vi "Halvorsen_Euler_Fast.vi"(0 "tolerance":dbl=1e-13, 1 "Error Analysis":u16(ring)=4 items=["Max", "Max_Norm", "Norm", "Last Value", "Last Constant"], 3 "Шаг h, с":dbl=0.01, 4 "k":i32=8, 5 "Время, с":dbl=30.0, 7 "Hmax":dbl=1.0, 8 "Parameters":dbl[](array[numeric])=[1.4, 1.4, 1.4], 10 "last_point_Thomas":dbl[](array[numeric])=[2.3727475682665875, 0.23609824454436878, 0.4447912442126299], 13 "Hmin":dbl=0.001, 15 "Points count":i32=2, 18 "n":i32[](array[numeric])=[1, 2, 3, 4, 5, 6, 7, 8, 18, 20, 22], 19 "Ext.Type":u16(ring) items=["FNode", "MathScript", "ECD8 Arrays", "ECD8 Fnode", "ECD8 FnodeDiv", "FNode Exp"]) -> (6 "Elapsed Time":dbl=0.8335924918947057, 12 "Number of steps":i32=29504, 14 "Error Estimation":dbl=9.972073185504694, 17 "Rejected steps":i32=56)   [LabVIEW 2016]
uses:
  <vilib>/Analysis/_algsub.llb/Real Vector Norm.vi
  <vilib>/Analysis/5stat.llb/RMS (DBL).vi
  <vilib>/Analysis/NI_AALBase.lvlib
  <vilib>/Analysis/NI_AALPro.lvlib
panel:
  in  "Initial Conditions":dbl[](array[numeric])=[1.0, 0.0, 1.0]
  out "Last Value Reference":dbl[](array[numeric])=[-8.132376937433255, -1.7681295405184005, -0.1250130264252919] format="%#_15f"
  out "Rejected Steps":i32[](graph)
  out "Last Value":dbl[](array[numeric])=[-7.1287069315310125, 0.8112482175083243, -2.527381111815407] format="%#_16f"
  out "Step time variation":dbl[](graph)=[0.8416094721687841, 0.8255755116206274]
  out "Real Error":dbl[][](graph)
  out "Step Variation":dbl[](graph)
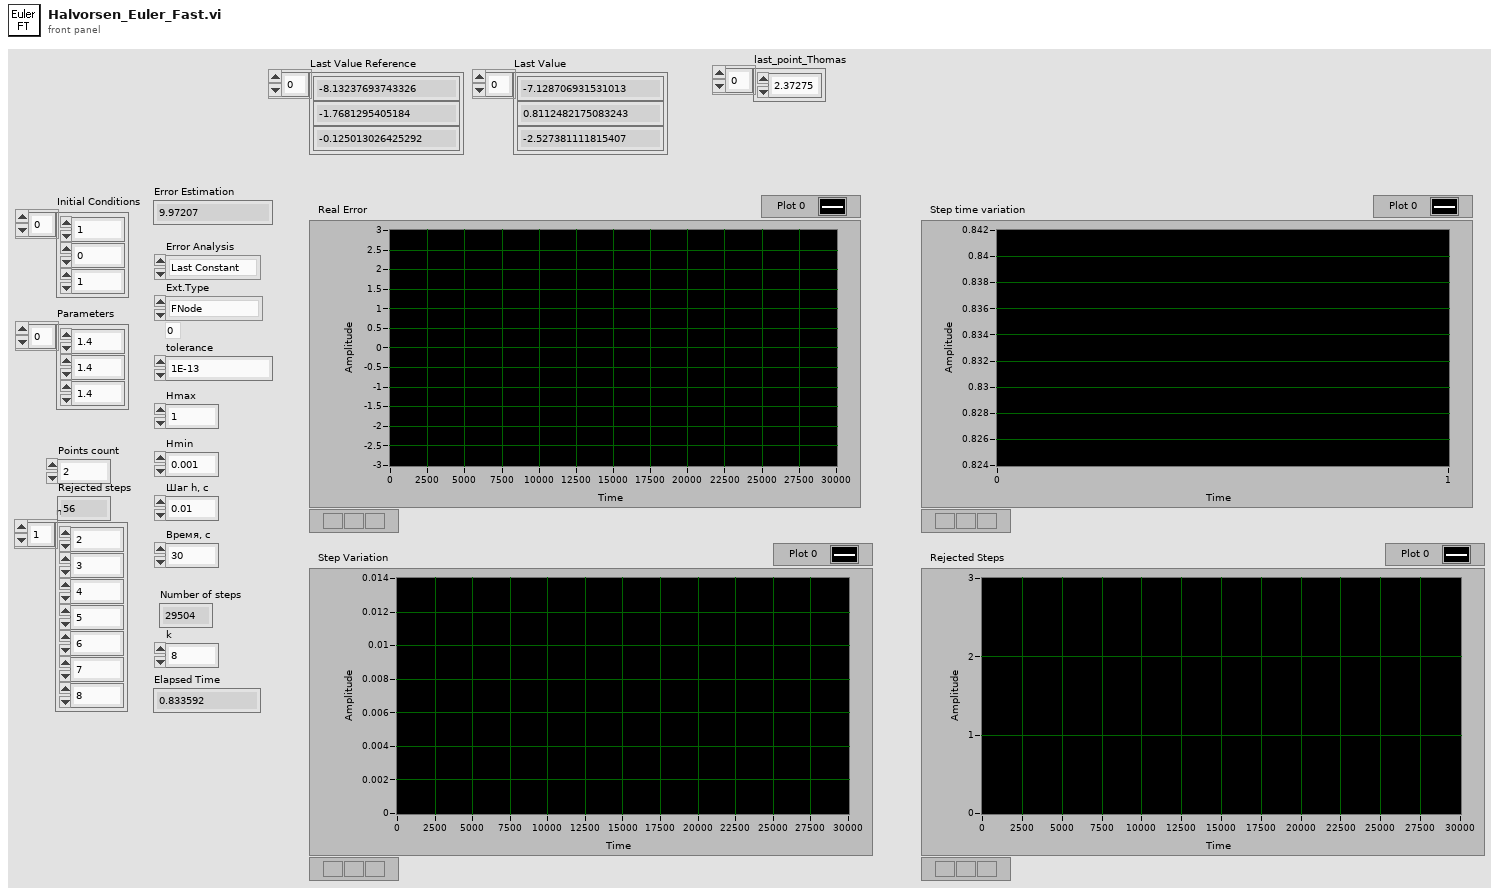
[diagram p1: front panel]
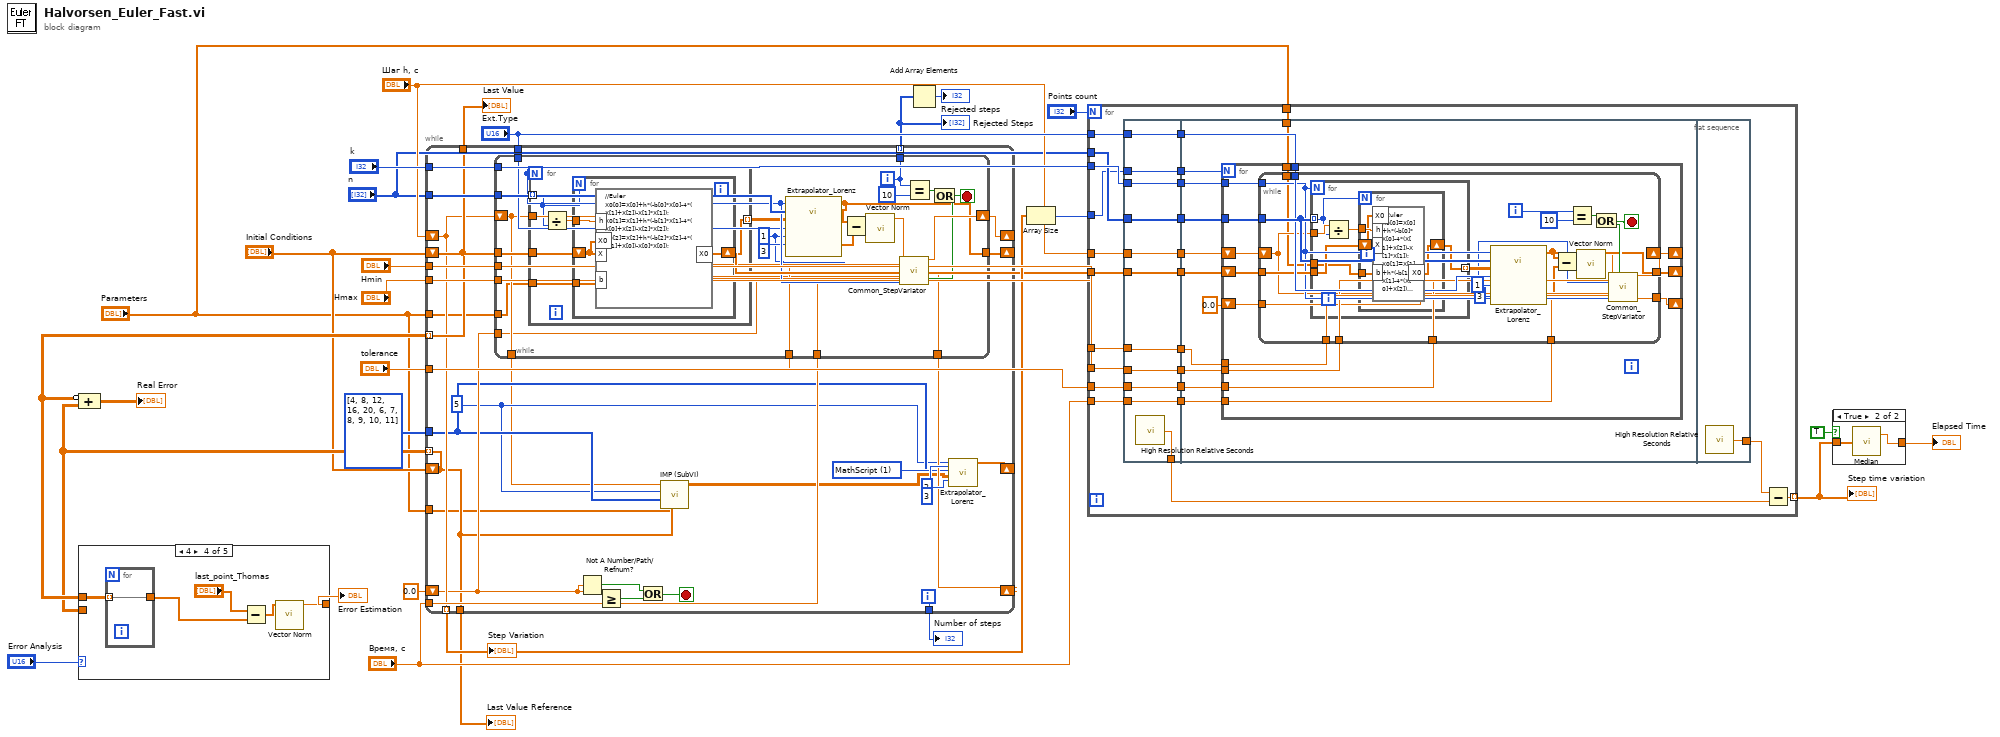
[diagram p0: block diagram]
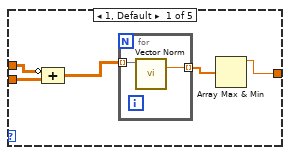
[diagram p2: hidden frame]
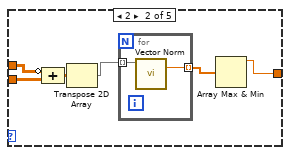
[diagram p3: hidden frame]
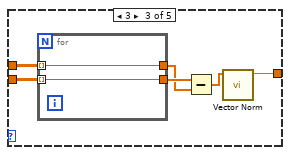
[diagram p4: hidden frame]
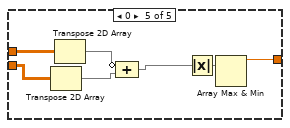
[diagram p5: hidden frame]
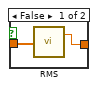
[diagram p6: hidden frame]
diagram:
  n1 = while {
    shift-right: [w50] -> _
    shift-left: "Initial Conditions" -> [w43]
    tunnel: "n" -> [w57]
    tunnel: "k" -> [w55]
    tunnel: "Ext.Type" -> [w46]
    shift-right: [w54] -> _
    shift-left: "Шаг h, с" -> [w37]
    shift-right: [w45] -> _
    shift-left: 0.0 -> [w36]
    tunnel: [w37] -> w13 mode=indexing
    tunnel: "Время, с" -> [w44]
    tunnel: [w56] -> w23
    tunnel: "tolerance" -> [w51]
    tunnel: "Hmin" -> [w53]
    tunnel: "Hmax" -> [w52]
    tunnel: [w43] -> w6 mode=indexing
    shift-right: [w49] -> _
    shift-left: "Initial Conditions" -> [w31]
    tunnel: i32[] [4, 8, 12, 16, 20, 6, 7, 8, 9, 10, 11] ("n 2") -> [w34]
    tunnel: [w31] -> w5 mode=indexing
    tunnel: [w43] -> w11
    tunnel: [w42] -> w10 mode=indexing
    tunnel: [w31] -> w4
    tunnel: "Parameters" -> [w35]
    tunnel: "Parameters" -> [w30]
    i -> [w56]
    stop <- w40 stop-if-true
    w41 = u16 1 items=["FNode", "MathScript", "ECD8 Arrays", "ECD8 Fnode", "ECD8 FnodeDiv"] ("Ext.Type")
    w33 = 5
    n2 = while {
      tunnel: w57 -> [w82]
      tunnel: w55 -> [w81]
      tunnel: w53 -> [w79]
      tunnel: w52 -> [w78]
      tunnel: w51 -> [w77]
      tunnel: [w60] -> w50
      tunnel: w46 -> [w74]
      tunnel: [w65] -> w45
      tunnel: w44 -> [w73]
      tunnel: w43 -> [w72]
      shift-right: [w80] -> w54
      shift-left: w37 -> [w67]
      tunnel: [w67] -> w32
      tunnel: [w66] -> w42
      tunnel: w36 -> [w64]
      tunnel: w35 -> [w62]
      i -> [w66]
      stop <- w69 stop-if-true
      w63 = 1 ("input variable")
      n3 = for {
        N: w81 -> [_]
        tunnel: w82 -> [w85] mode=indexing
        tunnel: w67 -> [w86]
        tunnel: w72 -> [w88]
        tunnel: [w87] -> w75 mode=indexing
        tunnel: w62 -> [w83]
        n4 = Divide(x=w86, y=w85) -> (x/y=w84:dbl)
        n5 = for {
          N: w85 -> [_]
          shift-right: [w92] -> w87
          shift-left: w88 -> [w90]
          tunnel: w84 -> [w91]
          tunnel: w83 -> [w89]
          n6 = formula code="//Euler\nX0[0]=X[0]+h*(-b[0]*X[0]-4*(X[1]+X[2])-X[1]*X[1]);\nX0[1]=X[1]+h*(-b[1]*X[1]-4*(X[0]+X[2])-X[2]*X[2]);\nX0[2]=X[2]+h*(-b[2]*X[2]-4*(X[1]+X[0])-X[0]*X[0]);"("X"=w90, "h"=w91, "X0"=w90, "b"=w89) -> ("X0"=w92:dbl[])
        }
      }
      n7 = call "Extrapolator_Lorenz.vi"("Порядок экстраполятора"=w63, "Dimension"=3 ("input variable"), "Ext.Type"=w74, "Х - нач. условия"=w75, "n"=w82, "k"=w81) -> ("TPrev"=w59:dbl[], "Tout"=w60:dbl[])  [unwired: 4 in]
      n8 = Subtract(x=w60, y=w59) -> (x-y=w61:dbl[])
      n9 = call-poly <vilib>:"Vector Norm.vi"("Input Vector"=w61) -> ("norm"=w58:dbl)  [unwired: 9 in, 1 out]
      n10 = call "Common_StepVariator.vi"("err"=w58, "tolerance"=w77, "Hmax"=w78, "Ord"=w63, "Шаг h, с"=w67, "Current time"=w64, "k"=w81, "Hmin"=w79, "tmax"=w73) -> ("Hnew"=w80:dbl, "New time"=w65:dbl, "stop"=w68:bool)  [unwired: 3 in, 1 out]
      n11 = Equal?(x=w66, y=10) -> (x = y?=w71:bool)
      n12 = Or(x=w71, y=w68) -> (x .or. y?=w69:bool)
    }
    n13 = Not A Number/Path/Refnum?(number/path/refnum=w36) -> (NaN/Path/Refnum?=w38:bool)
    n14 = Greater Or Equal?(x=w36, y=w44) -> (x >= y?=w39:bool)
    n15 = Or(x=w38, y=w39) -> (x .or. y?=w40:bool)
    n16 = call "IMP (SubVI).vi"("Initial Conditions in"=w31, "b"=w30, "n in"=w34, "Numeric"=w33, "Шаг h, с"=w32) -> ("Initial Conditions out"=w29:dbl[][])  [unwired: 6 in]
    n17 = call "Extrapolator_Lorenz.vi"("Порядок экстраполятора"=2, "Dimension"=3, "Ext.Type"=w41, "Х - нач. условия"=w29, "n"=w34, "k"=w33) -> ("Tout"=w49:dbl[])  [unwired: 4 in, 1 out]
  }
  "Step Variation" <- w13
  "Number of steps" <- w23
  "Last Value" <- w11
  "Rejected Steps" <- w10
  "Last Value Reference" <- w4
  n18 = Compound Arithmetic op=ADD(invert w6, w5) -> (→"Real Error":dbl[][])
  n19 = case shown="4" "Error Analysis" {
    tunnel: w5 -> [w94 w102 w111 _ w122]
    tunnel: [w96 w104 w113 w120 w127] -> w8
    tunnel: w6 -> [w95 w103 w112 w119 w123]
    frame 1, Default {
      n20 = Compound Arithmetic op=ADD(invert w95, w94) -> (w93:dbl[][])
      n21 = for {
        tunnel: [w99] -> w97 mode=indexing
        tunnel: w93 -> [w98] mode=indexing
        n22 = call-poly <vilib>:"Vector Norm.vi"("Input Vector"=w98) -> ("norm"=w99:dbl)  [unwired: 9 in, 1 out]
      }
      n23 = Array Max & Min(array=w97) -> (max value=w96:dbl)  [unwired: 3 out]
    }
    frame 2 {
      n24 = Compound Arithmetic op=ADD(invert w103, w102) -> (w101:dbl[][])
      n25 = Transpose 2D Array(2D array=w101) -> (transposed array=w100:dbl[][])
      n26 = for {
        tunnel: [w107] -> w105 mode=indexing
        tunnel: w100 -> [w106] mode=indexing
        n27 = call-poly <vilib>:"Vector Norm.vi"("Input Vector"=w106) -> ("norm"=w107:dbl)  [unwired: 9 in, 1 out]
      }
      n28 = Array Max & Min(array=w105) -> (max value=w104:dbl)  [unwired: 3 out]
    }
    frame 3 {
      n29 = for {
        tunnel: w112 -> [w115] mode=indexing
        tunnel: [w115] -> w109
        tunnel: w111 -> [w114] mode=indexing
        tunnel: [w114] -> w110
      }
      n30 = Subtract(x=w110, y=w109) -> (x-y=w108:dbl[])
      n31 = call-poly <vilib>:"Vector Norm.vi"("Input Vector"=w108) -> ("norm"=w113:dbl)  [unwired: 9 in, 1 out]
    }
    frame 4 {
      n32 = for {
        tunnel: w119 -> [w121] mode=indexing
        tunnel: [w121] -> w118
      }
      n33 = Subtract(x="last_point_Thomas", y=w118) -> (x-y=w117:dbl[])
      n34 = call-poly <vilib>:"Vector Norm.vi"("Input Vector"=w117) -> ("norm"=w120:dbl)  [unwired: 9 in, 1 out]
    }
    frame 0 {
      n35 = Transpose 2D Array(2D array=w122) -> (transposed array=w125:dbl[][])
      n36 = Transpose 2D Array(2D array=w123) -> (transposed array=w126:dbl[][])
      n37 = Compound Arithmetic op=ADD(invert w126, w125) -> (w124:dbl[][])
      n38 = Absolute Value(x=w124) -> (abs(x)=w128:dbl[][])
      n39 = Array Max & Min(array=w128) -> (max value=w127:dbl)  [unwired: 3 out]
    }
  }
  "Error Estimation" <- w8
  n40 = Add Array Elements(numeric array=w10) -> (sum=→"Rejected steps":i32)
  n41 = Array Size(array=w13) -> (size(s)=w22:i32)
  n42 = for {
    N: "Points count" -> [_]
    tunnel: "k" -> [w152]
    tunnel: "n" -> [w151]
    tunnel: "Ext.Type" -> [w131]
    tunnel: "Initial Conditions" -> [w150]
    tunnel: w22 -> [w149]
    tunnel: [w142] -> w20 mode=indexing
    tunnel: "Шаг h, с" -> [w133]
    tunnel: "Hmin" -> [w141]
    tunnel: "Hmax" -> [w138]
    tunnel: "tolerance" -> [w137]
    tunnel: "Время, с" -> [w135]
    tunnel: "Parameters" -> [w129]
    n43 = flat-sequence {
      tunnel: w149 -> [w160]
      tunnel: w150 -> [w161]
      tunnel: w151 -> [w162]
      tunnel: w152 -> [w163]
      tunnel: [w163] -> w148
      tunnel: [w162] -> w147
      tunnel: [w161] -> w146
      tunnel: [w160] -> w145
      tunnel: [w159] -> w143
      tunnel: w141 -> [w158]
      tunnel: [w158] -> w140
      tunnel: w138 -> [w157]
      tunnel: [w157] -> w139
      tunnel: w137 -> [w156]
      tunnel: [w156] -> w136
      tunnel: w135 -> [w155]
      tunnel: [w155] -> w134
      tunnel: w133 -> [w154]
      tunnel: [w154] -> w132
      tunnel: w131 -> [w153]
      tunnel: [w153] -> w130
      tunnel: w148 -> [w175]
      tunnel: w147 -> [w174]
      tunnel: w146 -> [w173]
      tunnel: w145 -> [w172]
      tunnel: w140 -> [w170]
      tunnel: w139 -> [w169]
      tunnel: w136 -> [w168]
      tunnel: w134 -> [w167]
      tunnel: w132 -> [w166]
      tunnel: w130 -> [w165]
      tunnel: w129 -> [w164]
      tunnel: [w225] -> w144
      frame #0 {
        n44 = call <vilib>:"High Resolution Relative Seconds.vi"() -> ("relative seconds"=w159:dbl)
      }
      frame #1 {
        n45 = for {
          N: w172 -> [_]
          shift-right: [w185] -> _
          shift-left: w173 -> [w187]
          tunnel: w174 -> [w189]
          tunnel: w175 -> [w184]
          tunnel: w165 -> [w188]
          shift-right: [w186] -> _
          shift-left: w166 -> [w179]
          tunnel: w170 -> [w183]
          tunnel: w169 -> [w182]
          tunnel: w168 -> [w181]
          shift-right: [w178] -> _
          shift-left: 0.0 -> [w177]
          tunnel: w167 -> [w180]
          tunnel: w164 -> [w176]
          n46 = while {
            tunnel: w189 -> [w214]
            tunnel: w188 -> [w213]
            tunnel: w187 -> [w212]
            tunnel: [w192] -> w185
            tunnel: w184 -> [w208]
            tunnel: w183 -> [w207]
            tunnel: w182 -> [w206]
            tunnel: w181 -> [w205]
            tunnel: w177 -> [w204]
            tunnel: w180 -> [w203]
            shift-right: [w209] -> w186
            shift-left: w179 -> [w196]
            tunnel: [w197] -> w178
            tunnel: w176 -> [w194]
            i -> [w199]
            stop <- w200 stop-if-true
            w195 = 1 ("input variable")
            n47 = for {
              N: w208 -> [_]
              tunnel: w214 -> [w217] mode=indexing
              tunnel: w196 -> [w218]
              tunnel: w212 -> [w220]
              tunnel: [w219] -> w210 mode=indexing
              tunnel: w194 -> [w215]
              n48 = Divide(x=w218, y=w217) -> (x/y=w216:dbl)
              n49 = for {
                N: w217 -> [_]
                shift-right: [w224] -> w219
                shift-left: w220 -> [w222]
                tunnel: w216 -> [w223]
                tunnel: w215 -> [w221]
                n50 = formula code="//Euler\nX0[0]=X[0]+h*(-b[0]*X[0]-4*(X[1]+X[2])-X[1]*X[1]);\nX0[1]=X[1]+h*(-b[1]*X[1]-4*(X[0]+X[2])-X[2]*X[2]);\nX0[2]=X[2]+h*(-b[2]*X[2]-4*(X[1]+X[0])-X[0]*X[0]);"("X"=w222, "h"=w223, "X0"=w222, "b"=w221) -> ("X0"=w224:dbl[])
              }
            }
            n51 = call "Extrapolator_Lorenz.vi"("Порядок экстраполятора"=w195, "Dimension"=3 ("input variable"), "Ext.Type"=w213, "Х - нач. условия"=w210, "n"=w214, "k"=w208) -> ("TPrev"=w191:dbl[], "Tout"=w192:dbl[])  [unwired: 4 in]
            n52 = Subtract(x=w192, y=w191) -> (x-y=w193:dbl[])
            n53 = Equal?(x=w199, y=10) -> (x = y?=w201:bool)
            n54 = call-poly <vilib>:"Vector Norm.vi"("Input Vector"=w193) -> ("norm"=w190:dbl)  [unwired: 9 in, 1 out]
            n55 = call "Common_StepVariator.vi"("err"=w190, "tolerance"=w205, "Hmax"=w206, "Ord"=w195, "Шаг h, с"=w196, "Current time"=w204, "k"=w208, "Hmin"=w207, "tmax"=w203) -> ("Hnew"=w209:dbl, "New time"=w197:dbl, "stop"=w198:bool)  [unwired: 3 in, 1 out]
            n56 = Or(x=w201, y=w198) -> (x .or. y?=w200:bool)
          }
        }
      }
      frame #2 {
        n57 = call <vilib>:"High Resolution Relative Seconds.vi"() -> ("relative seconds"=w225:dbl)
      }
    }
    n58 = Subtract(x=w144, y=w143) -> (x-y=w142:dbl)
  }
  "Step time variation" <- w20
  n59 = case shown="True" TRUE {
    tunnel: w20 -> [w226 w229]
    tunnel: [w227 w228] -> w19
    frame False {
      n60 = call-poly <vilib>:"RMS.vi"("X"=w226) -> ("rms value"=w227:dbl)  [unwired: 1 out]
    }
    frame True {
      n61 = call <vilib>:"Median.vi"("X"=w229) -> ("median"=w228:dbl)  [unwired: 1 out]
    }
  }
  "Elapsed Time" <- w19
